vi "Stream Menu Updates.vi"(8 "error in (no error)":errorcluster, 11 "Terminal Menus in":refnum<class "Terminal Menus.lvclass">) -> (0 "error out":errorcluster, 3 "Terminal Menus out":refnum<class "Terminal Menus.lvclass">)   [LabVIEW 2016, in "CLD Exam - ATM.lvlib" / "Terminal Menus.lvclass"]
uses:
  Terminal Menus.lvclass
  D:/Repos/Stream/software/Mediator/Classes/Mediated Actor/Mediated Actor.lvclass
  Mediator/Classes/Message String/Message String.lvclass
  D:/Repos/Stream/software/Mediator/Classes/Message Interface/Message Interface.lvclass
  Log/Application Log/Log Level.ctl
  Terminal Menus.lvclass/Terminal Menus.ctl
  Mediator/Classes/Message Transport Queue/Message Transport Queue.lvclass
  D:/Repos/Stream/software/Mediator/Classes/Message Transport Interface/Message Transport Interface.lvclass
  Mediator/Classes/Mediated Actor/Mediated Actor.lvclass
  Log/Application Log/Application Log.lvclass
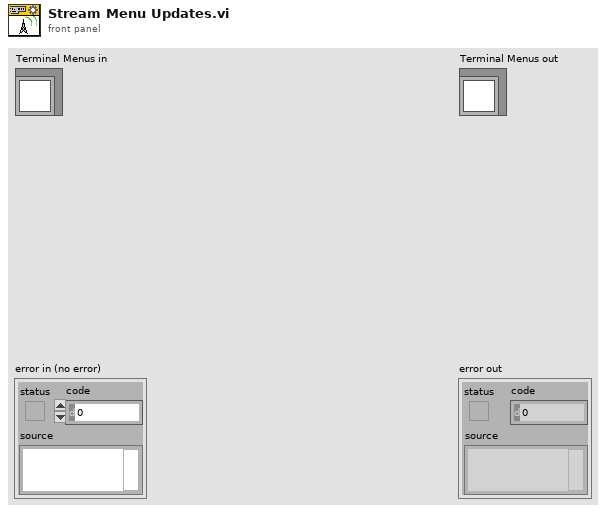
[diagram p1: front panel]
types:
  T1 = typedef "Stream Log.lvlib/Application Log.lvclass/Log Level.ctl" = enum16{"Imperative", "Major", "Minor", "Debug", "Off"}
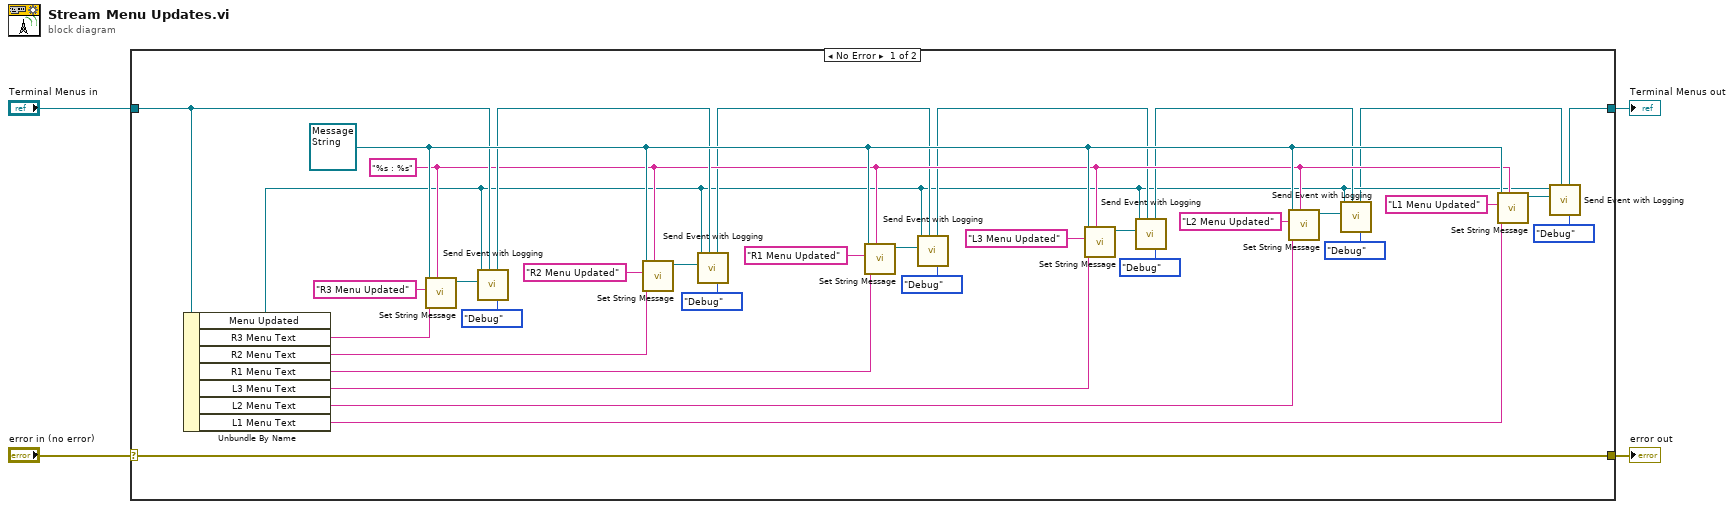
[diagram p0: block diagram]
diagram:
  n1 = case shown="No Error" "error in (no error)" {
    selector: "error in (no error)" -> [w39 w41]
    tunnel: [w39 w41] -> w3
    tunnel: [w5 w40] -> w1
    tunnel: "Terminal Menus in" -> [w23 w40]
    frame No Error {
      w19 = "%s : %s" ("Format")
      w26 = refnum<class "Message String.lvclass"> refnum ("Message String in")
      n2 = Unbundle By Name(w23) -> ("Menu Updated"=w7:refnum<class "Message Transport Queue.lvclass">, "R3 Menu Text"=w27:string, "R2 Menu Text"=w28:string, "R1 Menu Text"=w29:string, "L3 Menu Text"=w33:string, "L2 Menu Text"=w34:string, "L1 Menu Text"=w37:string)
      n3 = call "Set String Message.vi"("Format"=w19, "Value"=w27, "Name"="R3 Menu Updated", "Message String in"=w26) -> ("Message String out"=w24:refnum<class "Message String.lvclass">)  [unwired: 6 in, 1 out]
      n4 = call "Send Event with Logging.vi"("Global Log Level"=Log_Level."Debug", "Mediated Actor in"=w23, "Message"=w24, "Message Transport Interface in"=w7) -> ("Mediated Actor out"=w20:refnum<class "Terminal Menus.lvclass">)  [unwired: 6 in, 1 out]
      n5 = call "Set String Message.vi"("Format"=w19, "Value"=w28, "Name"="R2 Menu Updated", "Message String in"=w26) -> ("Message String out"=w21:refnum<class "Message String.lvclass">)  [unwired: 6 in, 1 out]
      n6 = call "Send Event with Logging.vi"("Global Log Level"=Log_Level."Debug", "Mediated Actor in"=w20, "Message"=w21, "Message Transport Interface in"=w7) -> ("Mediated Actor out"=w16:refnum<class "Terminal Menus.lvclass">)  [unwired: 6 in, 1 out]
      n7 = call "Set String Message.vi"("Format"=w19, "Value"=w29, "Name"="R1 Menu Updated", "Message String in"=w26) -> ("Message String out"=w17:refnum<class "Message String.lvclass">)  [unwired: 6 in, 1 out]
      n8 = call "Send Event with Logging.vi"("Global Log Level"=Log_Level."Debug", "Mediated Actor in"=w16, "Message"=w17, "Message Transport Interface in"=w7) -> ("Mediated Actor out"=w13:refnum<class "Terminal Menus.lvclass">)  [unwired: 6 in, 1 out]
      n9 = call "Set String Message.vi"("Format"=w19, "Value"=w33, "Name"="L3 Menu Updated", "Message String in"=w26) -> ("Message String out"=w14:refnum<class "Message String.lvclass">)  [unwired: 6 in, 1 out]
      n10 = call "Send Event with Logging.vi"("Global Log Level"=Log_Level."Debug", "Mediated Actor in"=w13, "Message"=w14, "Message Transport Interface in"=w7) -> ("Mediated Actor out"=w10:refnum<class "Terminal Menus.lvclass">)  [unwired: 6 in, 1 out]
      n11 = call "Set String Message.vi"("Format"=w19, "Value"=w34, "Name"="L2 Menu Updated", "Message String in"=w26) -> ("Message String out"=w11:refnum<class "Message String.lvclass">)  [unwired: 6 in, 1 out]
      n12 = call "Send Event with Logging.vi"("Global Log Level"=Log_Level."Debug", "Mediated Actor in"=w10, "Message"=w11, "Message Transport Interface in"=w7) -> ("Mediated Actor out"=w6:refnum<class "Terminal Menus.lvclass">)  [unwired: 6 in, 1 out]
      n13 = call "Set String Message.vi"("Format"=w19, "Value"=w37, "Name"="L1 Menu Updated", "Message String in"=w26) -> ("Message String out"=w8:refnum<class "Message String.lvclass">)  [unwired: 6 in, 1 out]
      n14 = call "Send Event with Logging.vi"("Global Log Level"=Log_Level."Debug", "Mediated Actor in"=w6, "Message"=w8, "Message Transport Interface in"=w7) -> ("Mediated Actor out"=w5:refnum<class "Terminal Menus.lvclass">)  [unwired: 6 in, 1 out]
    }
    frame Error {
    }
  }
  "error out" <- w3
  "Terminal Menus out" <- w1
